vi "Mail.vi"(1 "Contenue":string, 2 "Subject":string) -> ()   [LabVIEW 2022 SP3]
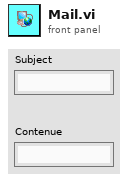
[diagram p1: front panel]
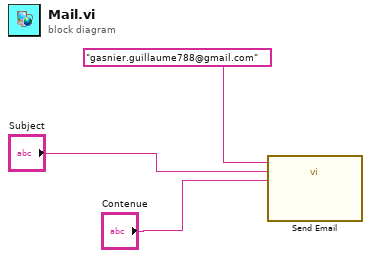
[diagram p0: block diagram]
diagram:
  n1 = call "Send Email"("Message"="Contenue", "Subject"="Subject", "Recipients"="gasnier.guillaume788@gmail.com") -> ()  [unwired: 8 in, 1 out]
